vi "dome_checkCallbacks.vi"(8 "error in (no error)":errorcluster) -> (0 "error out":errorcluster)   [LabVIEW 2015, in "SALLV_dome.lvlib"]
doc: "void dome_shm_checkCallbacksLV();"
uses:
  SALLV_dome.lvlib
  SALLV_dome.so
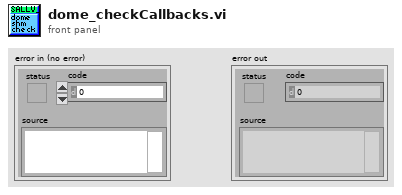
[diagram p1: front panel]
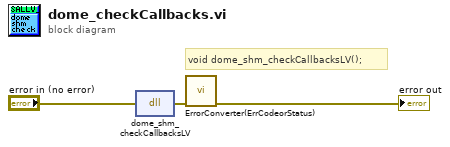
[diagram p0: block diagram]
diagram:
  # "void dome_shm_checkCallbacksLV();"
  n1 = dll-call lib="home/andres/Desktop/SALLV_dome2015/SALLV_dome.*" fn="dome_shm_checkCallbacksLV"(error in="error in (no error)") -> (error out=w2:errorcluster)  [unwired: 3 in, 1 out]
  n2 = call "ErrorConverter(ErrCodeorStatus).vi"("error in (no error)"=w2) -> ("error out"=→"error out":errorcluster)  [unwired: 10 in]
